vi "WPI_SerialPortOpen_USB.vi"(0 "Baud Rate":u32=9600, 1 "Timeout Value (ms)":u32=5000, 2 "Termination Char (0xA = '\\n' = LF)":u8=10 format="%.0x", 3 "Enable Termination Char? (T)":bool=TRUE, 5 "Data Bits":u16=8, 7 "Parity":u16(ring) items=["None", "Odd", "Even", "Mark", "Space"], 9 "Stop Bits":u16(ring)=10 items=["1.0"=10, "1.5"=15, "2.0"=20], 11 "error in (no error)":errorcluster, 12 "Flow Control":u16(ring) items=["None", "XON/XOFF", "RTS/CTS", "XON/XOFF & RTS/CTS", "DTR/DSR", "XON/XOFF & DTR/DSR"], 13 "Serial Port":T1=enum."MXP TTL") -> (4 "SerialPortRef":T2, 15 "error out":errorcluster)   [LabVIEW 2016, in "_NI WPI Serial USB.lvlib"]
doc: "Opens a reference to the serial port. You must open a reference before using any other VIs on this palette.\n\nThis software is licensed. Open the labview\\readme\\WPI Robotics Library Open Source License.txt file for more information."
uses:
  _NI WPI Serial USB.lvlib
  <vilib>/Rock Robotics/WPI/SerialPort/WPI_SerialPortRef.ctl
  WPI_SerialPort_USB.ctl
  <vilib>/Rock Robotics/SystemInterfaces/NetworkCommunication/NetComm_UsageReport_ResourceType.ctl
  <vilib>/Instr/_visa.llb/VISA Configure Serial Port (Instr).vi
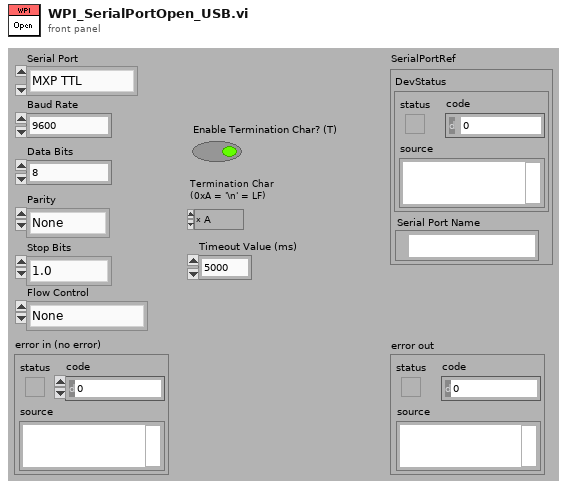
[diagram p1: front panel]
types:
  T1 = typedef "_NI WPI Serial USB.lvlib/WPI_SerialPort_USB.ctl" = enum16{"Onboard RS-232", "MXP TTL", "USB"}
  T2 = typedef "WPI_SerialPortRef.ctl" = cluster{"DevStatus":errorcluster, "Serial Port Name":refnum<visa-resource-name>}
  T3 = typedef "NetComm_UsageReport_ResourceType.ctl" = enum8{"Controller", "Module", "Language", "CANPlugin", "Accelerometer", "ADXL345", "AnalogChannel", "AnalogTrigger", "AnalogTriggerOutput", "CANJaguar", "Compressor", "Counter", "Dashboard", "DigitalInput", "DigitalOutput", "DriverStationCIO", "DriverStationEIO", "DriverStationLCD", "Encoder", "GearTooth", "Gyro", "I2C", "Framework", "Jaguar", "Joystick", "Kinect", "KinectStick", "PIDController", "Preferences", "PWM", "Relay", "RobotDrive", "SerialPort", "Servo", "Solenoid", "SPI", "Task", "Ultrasonic", "Victor", "Button", "Command", "AxisCamera", "PCVideoServer", "SmartDashboard", "Talon", "HiTechnicColorSensor", "HiTechnicAccel", "HiTechnicCompass", "SRF08", "AnalogOutput", "Victor SP", "Talon SRX", "CAN Talon SRX", "ADXL362 Accel", "ADXRS450 Gyro", "Rev SPARK", "Mindsensors SD540", "Digital Filter"}
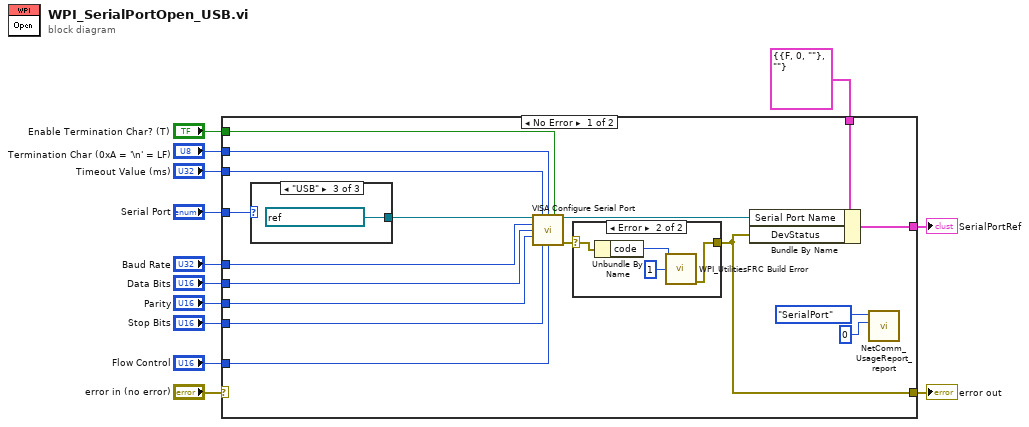
[diagram p0: block diagram]
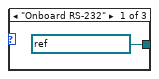
[diagram p2: hidden frame]
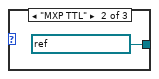
[diagram p3: hidden frame]
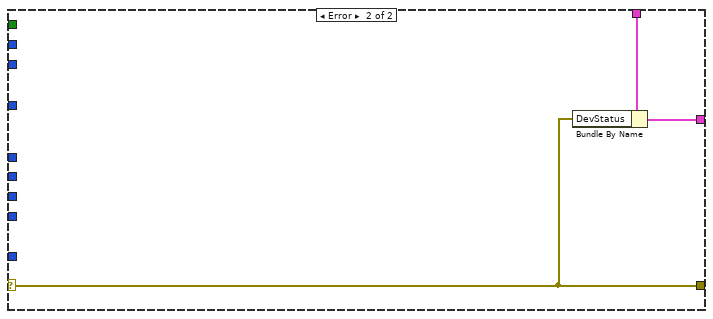
[diagram p5: hidden frame]
diagram:
  n1 = case shown="No Error" "error in (no error)" {
    selector: "error in (no error)" -> [_ w40]
    tunnel: "Baud Rate" -> [w26 _]
    tunnel: "Parity" -> [w24 _]
    tunnel: "Data Bits" -> [w25 _]
    tunnel: [w19 w41] -> w10
    tunnel: "Stop Bits" -> [w17 _]
    tunnel: [w16 w40] -> w7
    tunnel: T2 {"DevStatus"={"status"=FALSE, "code"=0, "source"=""}, "Serial Port Name"=""} ("SerialPortRef") -> [w30 w39]
    tunnel: "Enable Termination Char? (T)" -> [w20 _]
    tunnel: "Termination Char (0xA = '\\n' = LF)" -> [w21 _]
    tunnel: "Timeout Value (ms)" -> [w15 _]
    tunnel: "Flow Control" -> [w18 _]
    tunnel: "Serial Port" -> [w27 _]
    frame No Error {
      n2 = case shown="\"USB\"" w27 {
        tunnel: [refnum<visa-resource-name> "ASRL1::INSTR" ("VISA resource name") refnum<visa-resource-name> "ASRL2::INSTR" ("VISA resource name") refnum<visa-resource-name> "ASRL3::INSTR" ("VISA resource name")] -> w14
        frame "Onboard RS-232" {
        }
        frame "MXP TTL" {
        }
        frame "USB" {
        }
      }
      n3 = call-poly "VISA Configure Serial Port"("VISA resource name"=w14, "timeout (10sec)"=w15, "termination char\n(0xA = '\\n' = LF)"=w21, "Enable Termination\nChar (T)"=w20, "baud rate (9600)"=w26, "data bits (8)"=w25, "parity (0:none)"=w24, "stop bits (10: 1 bit)"=w17, "flow control (0:none)"=w18) -> ("VISA resource name out"=w23:refnum<visa-resource-name>, "error out"=w22:errorcluster)  [unwired: 5 in]
      n4 = case shown="Error" w22 {
        selector: w22 -> [w34 w36]
        tunnel: [w34 w35] -> w16
        frame No Error {
        }
        frame Error {
          n5 = Unbundle By Name(w36) -> ("code"=w38:i32)
          n6 = call <vilib>:"WPI_UtilitiesFRC Build Error.vi"("error code"=w38, "chain levels to remove (1)"=1) -> ("error out"=w35:errorcluster)  [unwired: 3 in, 10 out]
        }
      }
      n7 = Bundle By Name(cluster=w30, "Serial Port Name"=w23, "DevStatus"=w16) -> (w19:T2)
      n8 = call <vilib>:"NetComm_UsageReport_report.vi"("Instance Number"=u8 0, "Resource Type"=NetComm_UsageReport_ResourceType."SerialPort") -> ()  [unwired: 10 in]
    }
    frame Error {
      n9 = Bundle By Name(cluster=w39, "DevStatus"=w40) -> (w41:T2)
    }
  }
  "error out" <- w7
  "SerialPortRef" <- w10
